vi "I0.vi"(0 "Iscn":dbl, 1 "T":dbl, 2 "Vocn":dbl, 3 "KI":dbl, 4 "Tn":dbl, 5 "KV":dbl, 6 "ns":dbl, 8 "a":dbl=1.3) -> (7 "I0":dbl)   [LabVIEW 2016]
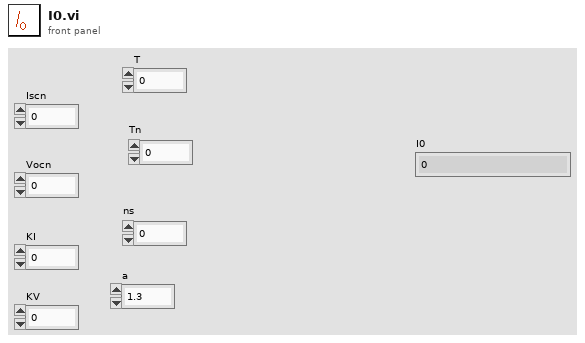
[diagram p1: front panel]
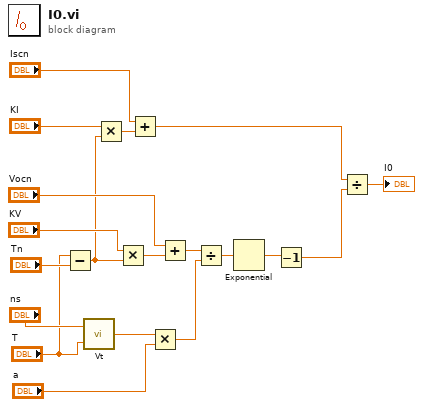
[diagram p0: block diagram]
diagram:
  n1 = Subtract(x="T", y="Tn") -> (x-y=w6:dbl)
  n2 = call "Vt.vi"("T"="T", "ns"="ns") -> ("Vt"=w18:dbl)
  n3 = Multiply(x="KI", y=w6) -> (x*y=w5:dbl)
  n4 = Multiply(x="KV", y=w6) -> (x*y=w12:dbl)
  n5 = Add(x="Iscn", y=w5) -> (x+y=w1:dbl)
  n6 = Multiply(x=w18, y="a") -> (x*y=w10:dbl)
  n7 = Add(x="Vocn", y=w12) -> (x+y=w11:dbl)
  n8 = Divide(x=w11, y=w10) -> (x/y=w9:dbl)
  n9 = Exponential(1:w9) -> (0:w8:dbl)
  n10 = Decrement(x=w8) -> (x-1=w2:dbl)
  n11 = Divide(x=w1, y=w2) -> (x/y=→"I0":dbl)
